vi "AdvFilter-Design.vi"(6 "order":i32=7, 7 "filter type":T2, 8 "Class":enum16{"Elliptic", "Butterworth"}(ring), 9 "low cutoff freq: fl":dbl=0.125 format="%0.3f", 10 "high cutoff freq: fh":dbl=0.45 format="%0.3f", 11 "sampling freq: fs":dbl=1.0 format="%0.2f") -> (0 "error":i32, 3 "IIR Filter":T1)   [LabVIEW 2020]
uses:
  <vilib>/Analysis/3filter.llb/Filter Passband Type.ctl
  <vilib>/Analysis/NI_AALBase.lvlib
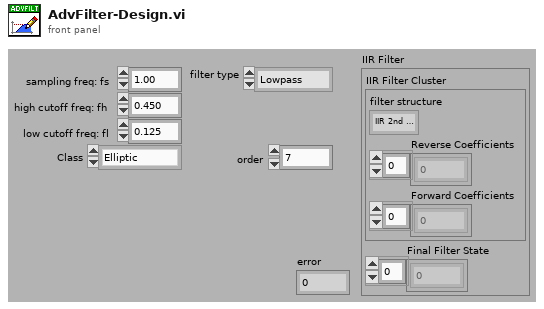
[diagram p1: front panel]
types:
  T1 = cluster{"IIR Filter Cluster":cluster{"filter structure":enum32{"IIR 2nd Order", "IIR 4th Order"}, "Reverse Coefficients":dbl[], "Forward Coefficients":dbl[]}, "Final Filter State":dbl[]}
  T2 = typedef "NI_AALBase.lvlib/Filter Passband Type.ctl" = enum32{"Lowpass", "Highpass", "Bandpass", "Bandstop"}
  T3 = cluster{"filter structure":enum32{"IIR 2nd Order", "IIR 4th Order"}, "Reverse Coefficients":dbl[], "Forward Coefficients":dbl[]}
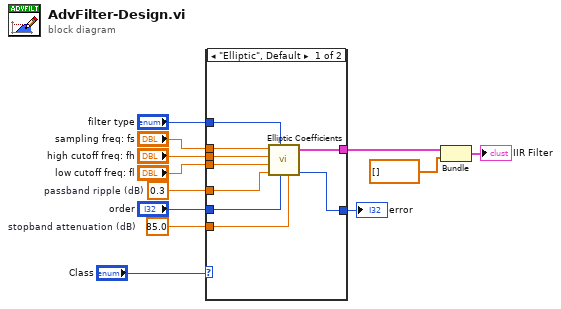
[diagram p0: block diagram]
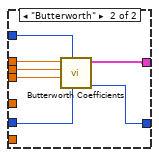
[diagram p2: hidden frame]
diagram:
  w10 = 85.0  # stopband attenuation (dB)
  w12 = 0.3  # passband ripple (dB)
  n1 = case shown="\"Elliptic\", Default" "Class" {
    tunnel: w12 -> [w21 _]
    tunnel: "order" -> [w20 w24]
    tunnel: w10 -> [w19 _]
    tunnel: "filter type" -> [w18 w27]
    tunnel: "sampling freq: fs" -> [w17 w28]
    tunnel: "high cutoff freq: fh" -> [w16 w26]
    tunnel: "low cutoff freq: fl" -> [w15 w25]
    tunnel: [w14 w23] -> w5
    tunnel: [w13 w22] -> w1
    frame "Elliptic", Default {
      n2 = call <vilib>:"Elliptic Coefficients.vi"("stopband attenuation (dB)"=w19, "order"=w20, "filter type"=w18, "passband ripple (dB)"=w21, "low cutoff freq: fl"=w15, "high cutoff freq: fh"=w16, "sampling freq: fs"=w17) -> ("error"=w13:i32, "IIR Filter Cluster"=w14:T3)  [unwired: 3 in]
    }
    frame "Butterworth" {
      n3 = call <vilib>:"Butterworth Coefficients.vi"("order"=w24, "filter type"=w27, "low cutoff freq: fl"=w25, "high cutoff freq: fh"=w26, "sampling freq: fs"=w28) -> ("error"=w22:i32, "IIR Filter Cluster"=w23:T3)  [unwired: 5 in]
    }
  }
  "error" <- w1
  n4 = Bundle("IIR Filter Cluster"=w5, "Final Filter State"=dbl[] []) -> (→"IIR Filter":T1)  [unwired: 1 in]
